vi "Generate Address Frame Vectors.vi"(0 "RFFE RegReadExt Command in":refnum<class "RFFE RegReadExt Command.lvclass">, 11 "error in (no error)":errorcluster) -> (4 "RFFE RegReadExt Command out":refnum<class "RFFE RegReadExt Command.lvclass">, 6 "Address Frame Vectors":string[](array[string]), 15 "error out":errorcluster)   [LabVIEW 2018, in "MIPI RFFE API.lvlib" / "RFFE RegReadExt Command.lvclass"]
uses:
  RFFE RegReadExt Command.lvclass
  Extended Command/RFFE Extended Command.lvclass
  MIPI RFFE API.lvlib
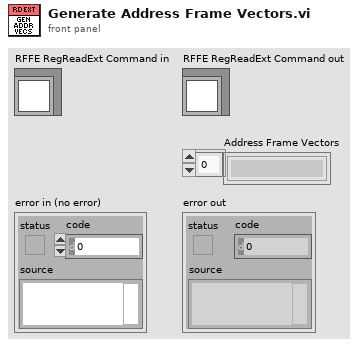
[diagram p1: front panel]
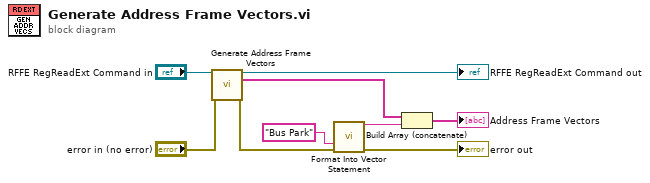
[diagram p0: block diagram]
diagram:
  n1 = call-parent "Generate Address Frame Vectors.vi"("RFFE Extended Command in"="RFFE RegReadExt Command in", "error in (no error)"="error in (no error)") -> ("RFFE Extended Command out"=→"RFFE RegReadExt Command out":refnum<class "RFFE RegReadExt Command.lvclass">, "Address Frame Vectors"=w6:string[], "error out"=w5:errorcluster)  [unwired: 11 in]
  n2 = call "Format Into Vector Statement.vi"("Comment"="Bus Park", "error in (no error)"=w5) -> ("Vector Statement"=w3:string, "error out"=→"error out":errorcluster)  [unwired: 12 in]
  n3 = Build Array (concatenate)(w6, w3) -> (→"Address Frame Vectors":string[])
